vi "Three 16-bit Ports Digital Output.vi"(2 "Packet":u64, 4 "Three 16-bit DO Ports":T1={"16-Bit DO Port0"="Chassis2/Mod2/DO15:0", "16-Bit DO Port1"="Chassis2/Mod2/DO15:0", "16-Bit DO Port3"="Chassis2/Mod2/DO15:0"}) -> ()   [LabVIEW 2009]
uses:
  <vilib>/eio/EIONode/EIONode.xnode
  <vilib>/rvi/eio/nirviEIOImplementation/nirviEIOImplementation.xnode
  <vilib>/rvi/eio/common/nirviEmuTemplateMethod_noerrors.vi
  <vilib>/rvi/eio/common/nirviEmuClasses.ctl
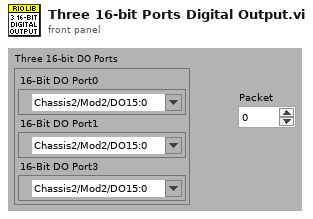
[diagram p1: front panel]
types:
  T1 = cluster{"16-Bit DO Port0":refnum<k21>, "16-Bit DO Port1":refnum<k21>, "16-Bit DO Port3":refnum<k21>}
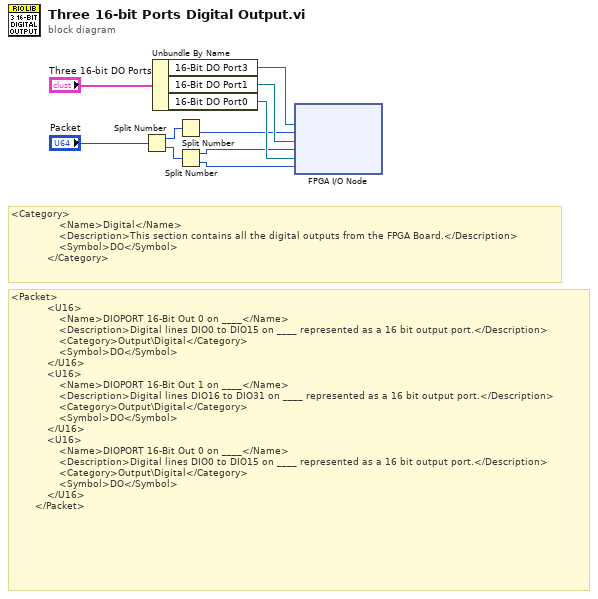
[diagram p0: block diagram]
diagram:
  # "<Packet>\n            <U16>\n                <Name>DIOPORT 16-Bit Out 0 on ____</Name>\n                <Description>Digital lines DIO0 to DIO15 on ____ represented as a 16 bit output port.</Description>\n                <Category>Output\\Digital</Category>\n                <Symbol>DO</Symbol>\n            </U16>\n            <U16>\n                <Name>DIOPORT 16-Bit Out 1 on ____</Name>\n                <Description>Digital lines DIO16 to DIO31 on ____ represented as a 16 bit output port.</Description>\n                <Category>Output\\Digital</Category>\n                <Symbol>DO</Symbol>\n            </U16>\n            <U16>\n                <Name>DIOPORT 16-Bit Out 0 on ____</Name>\n                <Description>Digital lines DIO0 to DIO15 on ____ represented as a 16 bit output port.</Description>\n                <Category>Output\\Digital</Category>\n                <Symbol>DO</Symbol>\n            </U16>\n        </Packet>"
  # "<Category>\n                <Name>Digital</Name>\n                <Description>This section contains all the digital outputs from the FPGA Board.</Description>\n                <Symbol>DO</Symbol>\n            </Category>"
  n1 = Split Number(x="Packet") -> (hi(x)=w2:u32, lo(x)=w10:u32)
  n2 = Unbundle By Name("Three 16-bit DO Ports") -> ("16-Bit DO Port3"=w3:refnum<k21>, "16-Bit DO Port1"=w7:refnum<k21>, "16-Bit DO Port0"=w6:refnum<k21>)
  n3 = Split Number(x=w2) -> (lo(x)=w1:u16)  [unwired: 1 out]
  n4 = Split Number(x=w10) -> (hi(x)=w5:u16, lo(x)=w4:u16)
  n5 = xnode "FPGA I/O Node"("I/O Item"=w1, "I/O Item"=w5, "I/O Item"=w4, "FPGA I/O In"=w3, "FPGA I/O In"=w7, "FPGA I/O In"=w6) -> ()  [unwired: 3 out]
